vi "CLD 5 Parse Config Data File.vi"(8 "Fehler (Eingang, kein Fehler)":errorcluster, 10 "Array (Eingang)":T1[][](array[typedef]), 11 "Abfragen/Festlegen":enum16{"Abfragen", "Festlegen"}(ring)) -> (0 "Fehler (Ausgang)":errorcluster, 3 "Array (Ausgang)":T1[][](array[typedef]))   [LabVIEW 2009]
doc: "CLD-Übung 5"
uses:
  CLD 5 Data Cluster.ctl
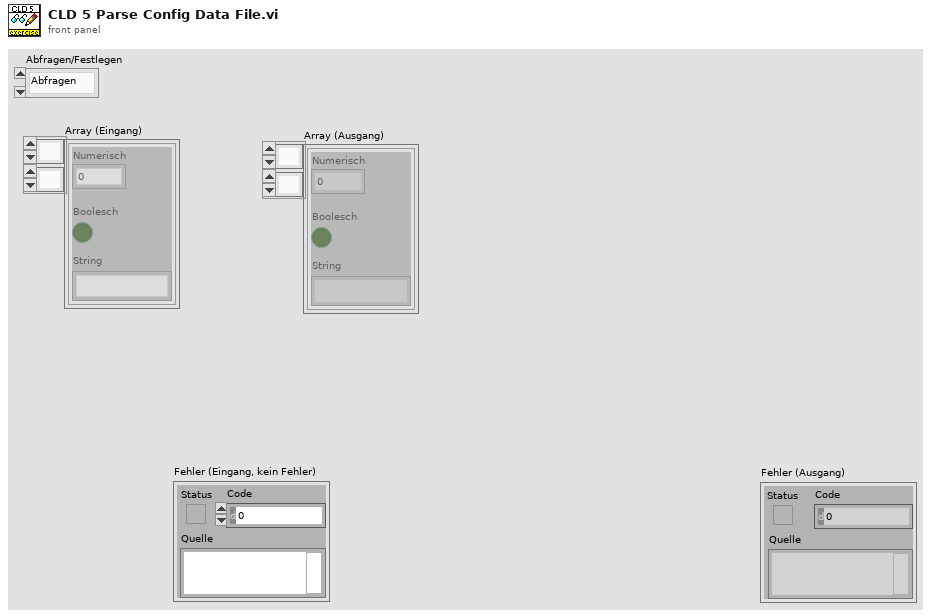
[diagram p1: front panel]
types:
  T1 = typedef "CLD 5 Data Cluster.ctl" = cluster{"Numerisch":dbl, "Boolesch":bool, "String":string}
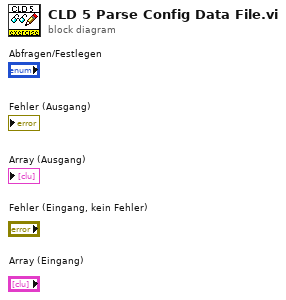
[diagram p0: block diagram]
diagram:
